vi "Temp_load_instr_data.vi"(3 "ParametresInstrumentaux":string[](array[string])) -> (0 "2e couple":string, 1 "1er couple":string, 2 "rayon":i32, 4 "champ":i32)   [LabVIEW 2010]
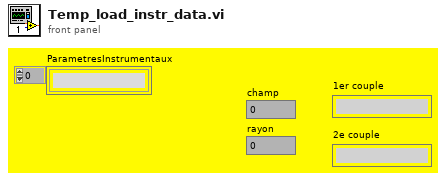
[diagram p1: front panel]
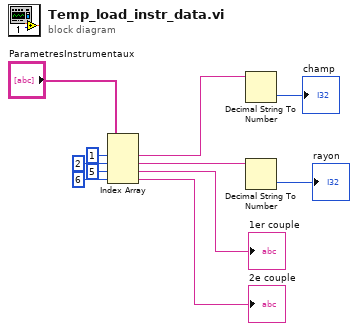
[diagram p0: block diagram]
diagram:
  n1 = Index Array(array="ParametresInstrumentaux", index #1=1 ("index"), index #2=2 ("index"), index #3=5 ("index"), index #4=6 ("index")) -> (element #1=w8:string, element #2=w7:string, element #3=→"1er couple":string, element #4=→"2e couple":string)
  n2 = Decimal String To Number(string=w8) -> (number=→"champ":i32)  [unwired: 2 in, 1 out]
  n3 = Decimal String To Number(string=w7) -> (number=→"rayon":i32)  [unwired: 2 in, 1 out]
